vi "LVObject Callback.vi"(8 "error in (no error)":errorcluster, 9 "Object Type":refnum<class>, 10 "Offset":i32, 11 "JSON String containing Flattened Object":string) -> (0 "error out":errorcluster, 1 "Object out":refnum<class>, 2 "Offset past match":i32)   [LabVIEW 2019]
uses:
  <userlib>/Blue Origin/BlueSerialization/BlueSerializer/BlueSerializer.lvclass
  StructuredData.ctl
  BlueJSONTextSerializer.lvclass
  OptionsFGVAction.ctl
  <vilib>/ErrorRing/Error Ring.xnode
  <vilib>/Utility/error.llb/Error Cluster From Error Code.vi
  C:/Program Files (x86)/National Instruments/LabVIEW 2019/user.lib/Blue Origin/BlueSerialization/BlueSerializer/BlueSerializer.lvclass
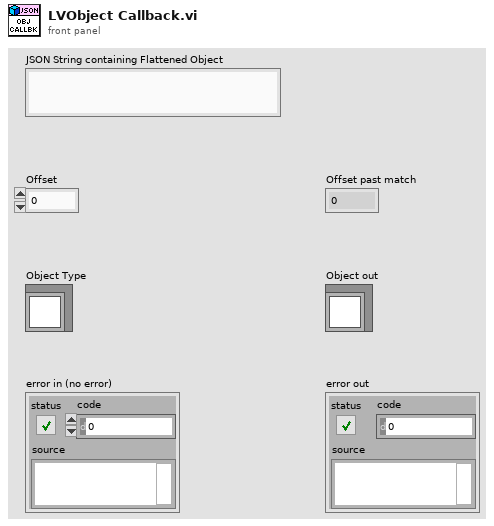
[diagram p1: front panel]
types:
  T1 = typedef "BlueJSONTextSerializer.lvlib/BlueJSONTextSerializer.lvclass/OptionsFGVAction.ctl" = enum16{"Remove", "Read", "Add"}
  T2 = typedef "BlueJSONTextSerializer.lvlib/BlueJSONTextSerializer.lvclass/StructuredData.ctl" = cluster{"JSON":string, "Offset":i32}
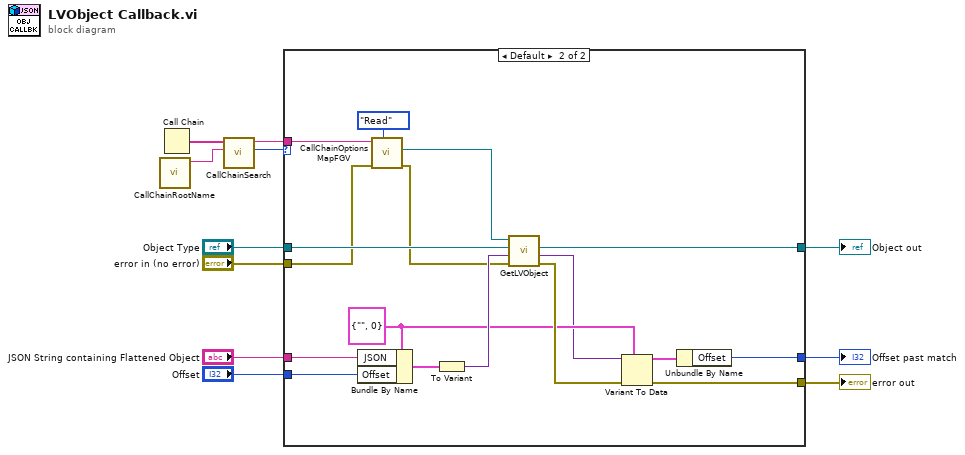
[diagram p0: block diagram]
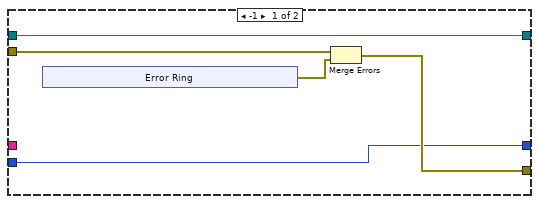
[diagram p2: hidden frame]
diagram:
  n1 = call "CallChainRootName.vi"() -> ("VI Name"=w5:string)  [unwired: 11 in]
  n2 = Call Chain() -> (call chain=w4:string[])
  n3 = call "CallChainSearch.vi"("Root VI name"=w5, "CallChain"=w4) -> ("Found index"=w1:i32, "Clone ID"=w3:string)  [unwired: 8 in]
  n4 = case shown="Default" w1 {
    tunnel: "JSON String containing Flattened Object" -> [_ w38]
    tunnel: "Offset" -> [w12 w37]
    tunnel: "Object Type" -> [w15 w36]
    tunnel: [w13 w32] -> w8
    tunnel: [w12 w29] -> w7
    tunnel: [w15 w28] -> w6
    tunnel: w3 -> [_ w27]
    tunnel: "error in (no error)" -> [w16 w25]
    frame -1 {
      n5 = xnode "Error Ring"() -> ("error out"=w14:errorcluster)
      n6 = Merge Errors(w16, w14) -> (w13:errorcluster)
    }
    frame Default {
      w31 = T2 {"JSON"="", "Offset"=0} ("Cluster")
      n7 = Bundle By Name(cluster=w31, "JSON"=w38, "Offset"=w37) -> (w35:T2)
      n8 = call "CallChainOptionsMapFGV.vi"("Action"=OptionsFGVAction."Read", "error in (no error)"=w25, "CloneID"=w27) -> ("error out"=w24:errorcluster, "BlueJSONTextSerializer (Read, Remove)"=w22:refnum<class "BlueJSONTextSerializer.lvclass">)  [unwired: 6 in, 1 out]
      n9 = To Variant(anything=w35) -> (Variant=w34:variant)
      n10 = call <userlib>:"GetLVObject.vi"("error in (no error)"=w24, "StructuredData in"=w34, "Object Type"=w36, "BlueSerializer in"=w22) -> ("error out"=w33:errorcluster, "StructuredData out"=w23:variant, "Object out"=w28:refnum<class>)  [unwired: 4 in, 1 out]
      n11 = Variant To Data(error in=w33, type=w31, Variant=w23) -> (data=w30:T2, error out=w32:errorcluster)
      n12 = Unbundle By Name(w30) -> ("Offset"=w29:i32)
    }
  }
  "error out" <- w8
  "Object out" <- w6
  "Offset past match" <- w7
